vi "Read stateAuto.vi"(8 "error in (no error)":errorcluster, 11 "StateAuto in":refnum<class "StateAuto.lvclass">) -> (0 "error out":errorcluster, 2 "Enum":T1, 3 "StateAuto out":refnum<class "StateAuto.lvclass">)   [LabVIEW 2017, in "StateAuto.lvclass"]
uses:
  StateAuto.lvclass
  controls/StateMachineAuto.ctl
  StateAuto.lvclass/StateAuto.ctl
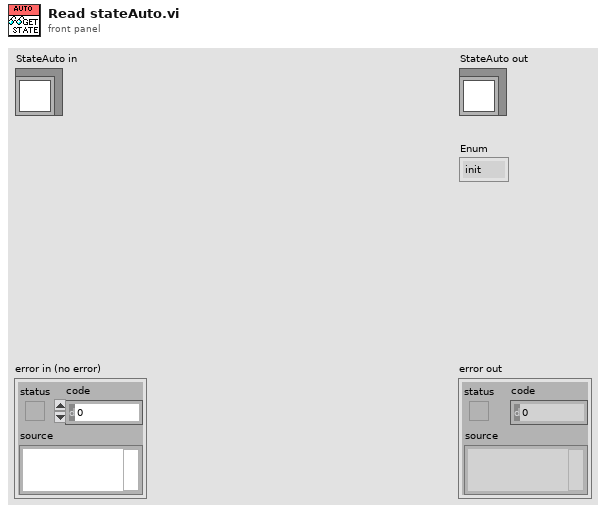
[diagram p1: front panel]
types:
  T1 = typedef "StateMachineAuto.ctl" = enum16{"init", "checkEMG", "checkStateBoard", "checkQueue", "writeDataQueue", "initNextCommand", "endNextCommand"}
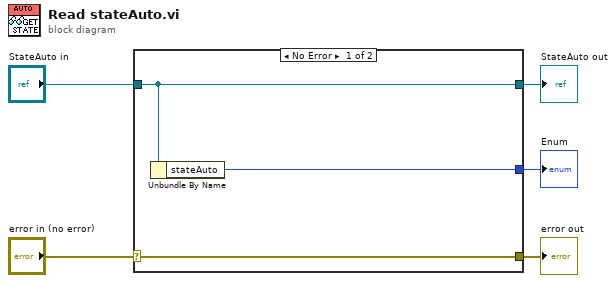
[diagram p0: block diagram]
diagram:
  n1 = case shown="No Error" "error in (no error)" {
    selector: "error in (no error)" -> [w8 w9]
    tunnel: [w8 w9] -> w4
    tunnel: [w7 w10] -> w2
    tunnel: "StateAuto in" -> [w7 w10]
    tunnel: [w6 _] -> w1
    frame No Error {
      n2 = Unbundle By Name(w7) -> ("stateAuto"=w6:T1)
    }
    frame Error {
    }
  }
  "error out" <- w4
  "StateAuto out" <- w2
  "Enum" <- w1
